vi "MVE Get Project Refnum.vi"(8 "error in (no error)":errorcluster, 10 "Full Path":string) -> (0 "error out":errorcluster, 3 "Project Refnum":refnum<vi>)   [LabVIEW 2016]
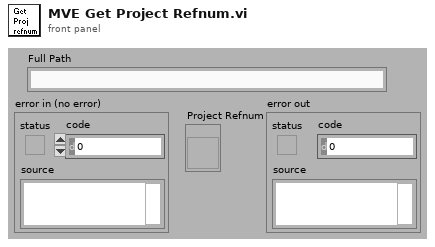
[diagram p1: front panel]
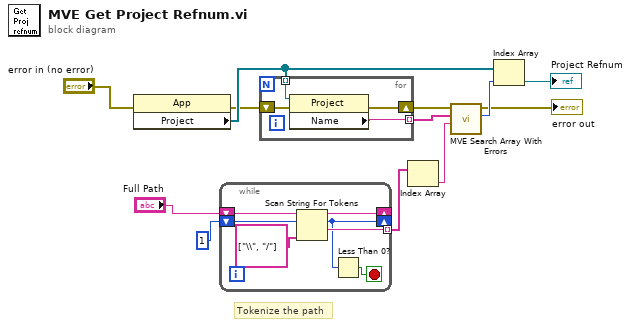
[diagram p0: block diagram]
diagram:
  # "Tokenize the path"
  n1 = property class="App"(error in="error in (no error)") -> (error out=w5:errorcluster, "Project"=w12:refnum<vi>[])  [unwired: 1 in, 1 out]
  n2 = while {
    tunnel: [w15] -> w8 mode=indexing
    shift-right: [w19] -> _
    shift-left: "Full Path" -> [w18]
    shift-right: [w13] -> _
    shift-left: 1 ("offset past token") -> [w17]
    stop <- w14 stop-if-true
    n3 = Scan String For Tokens(6:string[] ["\\", "/"] ("delimiters (\\s,\\t,\\r,\\n)"), 8:w17, 9:w18) -> (1:w15:string, 2:w13:i32, 3:w19:string)  [unwired: 3 in, 1 out]
    n4 = Less Than 0?(x=w13) -> (x < 0?=w14:bool)
  }
  n5 = for {
    tunnel: w12 -> [w23] mode=indexing
    tunnel: [w22] -> w2 mode=indexing
    shift-right: [w20] -> w3
    shift-left: w5 -> [w21]
    n6 = property class="Project"(reference=w23, error in=w21) -> (error out=w20:errorcluster, "Name"=w22:string)  [unwired: 1 out]
  }
  n7 = Index Array(array=w8) -> (element=w4:string)  [unwired: 1 in]
  n8 = call <resource>:"MVE Search Array With Errors.vi"("String"=w4, "Array of Strings"=w2, "error in (no error)"=w3) -> ("index of element"=w11:i32, "error out"=→"error out":errorcluster)  [unwired: 7 in]
  n9 = Index Array(array=w12, index=w11) -> (element=→"Project Refnum":refnum<vi>)
